vi "GyroTest.vi"() -> ()   [LabVIEW 2013]
panel:
  in  "Time Out (ms)":u32=1000
  in  "Stop Button":bool
  out "Angular displacement [LSB]":T1(graph)
  out "Angular rate [LSB/sec]":cluster{i16, i16, i16}(graph)
  in  "reset integrator":bool
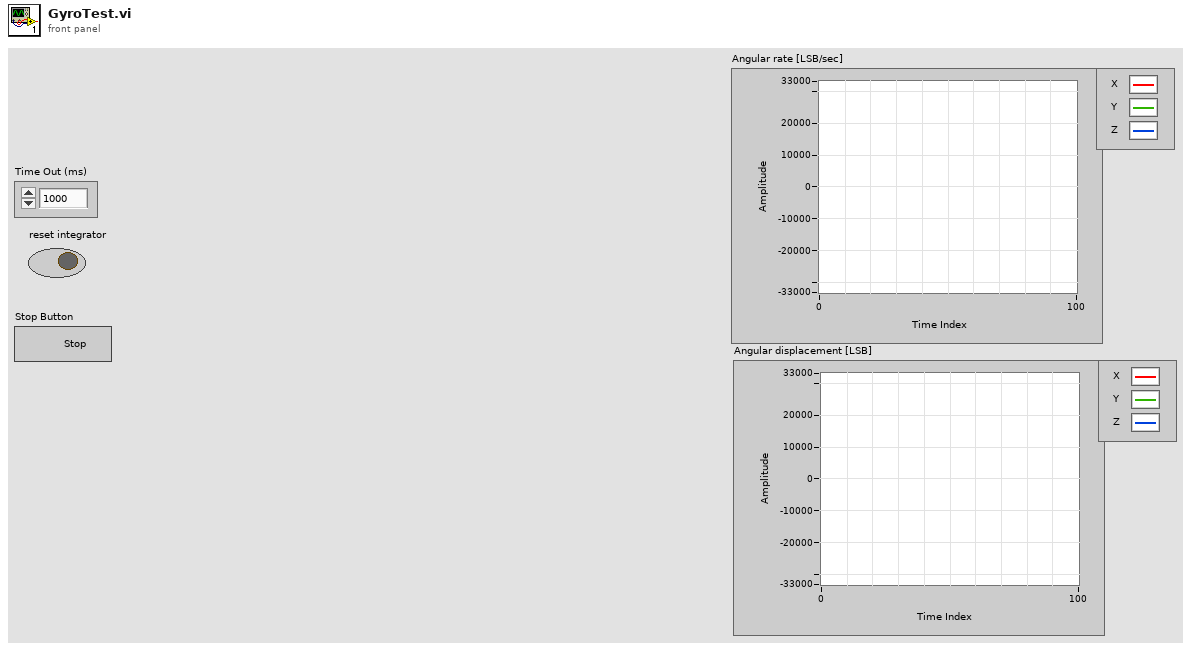
[diagram p1: front panel]
types:
  T1 = cluster{"integral x(t)":dbl, "integral x(t)":dbl, "integral x(t)":dbl}
  T2 = typedef "GyroReference.ctl" = cluster{"I2C Reference":T3, "DIO Reference":T11, "PmodGYRO address":u8}
  T3 = typedef "I2C.lvlib/I2C Reference.ctl" = cluster{"myRIO Reference":T4, "I2C Channels Enum":T8, "I2C Configuration":T9}
  T4 = typedef "myRIO Generic Hardware Reference.ctl" = cluster{"myRIO Model":T5, "myRIO Hardware Reference":T6}
  T5 = typedef "Hardware Version Enum.ctl" = enum16{"Unknown", "myRIO-1900", "myRIO-1950"}
  T6 = typedef "myRIO v1.0 Reference.ctl" = cluster{"Generic FPGA Reference":T7, "Allow multiple opens":bool}
  T7 = typedef "Generic FPGA Reference.ctl" = refnum<k20>
  T8 = typedef "I2C Channels Enum.ctl" = enum16{"Not Connected", "A/I2C", "B/I2C"}
  T9 = typedef "I2C.lvlib/I2C Configuration.ctl" = cluster{"I2C Transfer Rate":T10}
  T10 = typedef "I2C.lvlib/I2C Transfer Rate.ctl" = enum16{"Standard Mode (100 kbps)", "Fast Mode (400 kbps)"}
  T11 = typedef "DIO.lvlib/DIO Reference.ctl" = cluster{"myRIO Reference":T4, "DIO Channels List":T12}
  T12 = typedef "DIO Channels List.ctl" = T13[]
  T13 = typedef "DIO Channels Enum.ctl" = enum16{"Not Connected", "C/DIO0", "C/DIO1", "C/DIO2", "C/DIO3", "C/DIO4", "C/DIO5", "C/DIO6", "C/DIO7", "A/DIO0", "A/DIO1", "A/DIO2", "A/DIO3", "A/DIO4", "A/DIO5", "A/DIO6", "A/DIO7", "A/DIO8", "A/DIO9", "A/DIO10", "A/DIO11", "A/DIO12", "A/DIO13", "A/DIO14", "A/DIO15", "B/DIO0", "B/DIO1", "B/DIO2", "B/DIO3", "B/DIO4", "B/DIO5", "B/DIO6", "B/DIO7", "B/DIO8", "B/DIO9", "B/DIO10", "B/DIO11", "B/DIO12", "B/DIO13", "B/DIO14", "B/DIO15", "LED0", "LED1", "LED2", "LED3", "Button0"}
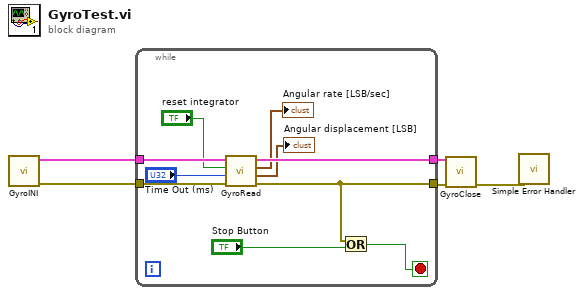
[diagram p0: block diagram]
diagram:
  n1 = call "GyroINI.vi"() -> ("Error Out"=w5:errorcluster, "GyroReference"=w4:T2)  [unwired: 10 in]
  n2 = while {
    tunnel: w5 -> [w14]
    tunnel: w4 -> [w15]
    tunnel: [w13] -> w3
    tunnel: [w9] -> w2
    stop <- w8 stop-if-true
    n3 = call "GyroRead.vi"("Error In"=w14, "Time Out (ms)"="Time Out (ms)", "reset integrator"="reset integrator", "GyroReference In"=w15) -> ("Error Out"=w9:errorcluster, "Angular displacement [LSB]"=→"Angular displacement [LSB]":T1, "Angular rate [LSB/sec]"=→"Angular rate [LSB/sec]":cluster{i16, i16, i16}, "GyroReference Out"=w13:T2)  [unwired: 3 in, 1 out]
    n4 = Or(x=w9, y="Stop Button") -> (x .or. y?=w8:bool)
  }
  n5 = call "GyroClose.vi"("Error In"=w2, "GyroReference In"=w3) -> ("Error Out"=w1:errorcluster)  [unwired: 9 in]
  n6 = call <vilib>:"Simple Error Handler.vi"("error in (no error)"=w1) -> ()  [unwired: 4 in, 5 out]
